vi "swerve.vi"(8 "POV Angle":i16=-1, 9 "Rotate Axis":dbl, 10 "Forwards Axis":dbl, 11 "Strafe Axis":dbl) -> (1 "Rotate Command":dbl, 2 "Forwards Command":dbl, 3 "Strafe Command":dbl)   [LabVIEW 2020]
panel:
  in  "POV Power":dbl=0.5
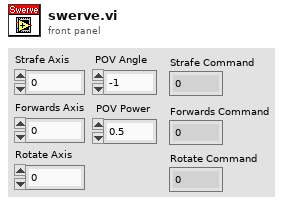
[diagram p1: front panel]
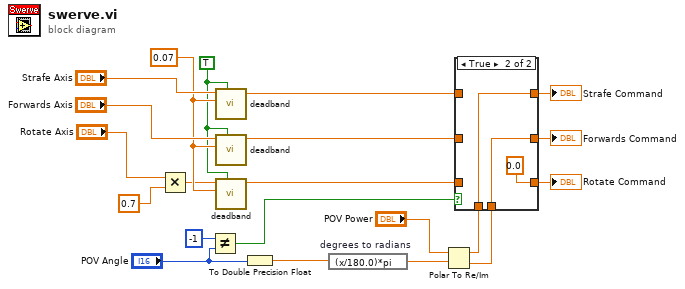
[diagram p0: block diagram]
diagram:
  w14 = 0.07 ("Deadband")
  w4 = TRUE ("Square Input?")
  n1 = Multiply(x="Rotate Axis", y=0.7) -> (x*y=w5:dbl)
  n2 = Not Equal?(x=i16 -1, y="POV Angle") -> (x != y?=w20:bool)
  n3 = call "deadband.vi"("Square Input?"=w4, "Deadband"=w14, "In"="Strafe Axis") -> ("Out"=w11:dbl)  [unwired: 8 in]
  n4 = call "deadband.vi"("Square Input?"=w4, "Deadband"=w14, "In"="Forwards Axis") -> ("Out"=w12:dbl)  [unwired: 8 in]
  n5 = call "deadband.vi"("Square Input?"=w4, "Deadband"=w14, "In"=w5) -> ("Out"=w13:dbl)  [unwired: 8 in]
  n6 = To Double Precision Float(number="POV Angle") -> (double precision float=w19:dbl)
  n7 = expression code="(x/180.0)*pi" "degrees to radians"(w19) -> (w7:dbl)
  n8 = Polar To Re/Im(2:w7, 3:"POV Power") -> (0:w10:dbl, 1:w9:dbl)
  n9 = case shown="True" w20 {
    tunnel: [w24 w27] -> w3
    tunnel: w9 -> [_ w27]
    tunnel: [w23 w26] -> w2
    tunnel: w10 -> [_ w26]
    tunnel: w11 -> [w24 _]
    tunnel: w12 -> [w23 _]
    tunnel: [w22 0.0 ("Out")] -> w1
    tunnel: w13 -> [w22 _]
    frame False {
    }
    frame True {
    }
  }
  "Strafe Command" <- w3
  "Forwards Command" <- w2
  "Rotate Command" <- w1
